vi "Send Command.vi"(7 "Config offset":u64 format="%x", 8 "error in (no error)":errorcluster, 9 "Command payload":u64 format="%x", 10 "Command number":T1, 11 "RP Instrument in":refnum<class "RP Instrument.lvclass">) -> (0 "error out":errorcluster, 3 "RP Instrument out":refnum<class "RP Instrument.lvclass">)   [LabVIEW 2016, in "RP Instrument.lvclass"]
uses:
  RP Instrument.lvclass
  RP Command.ctl
  RP Instrument.lvclass/RP Instrument.ctl
  RP Communicator/RP Communicator.lvclass
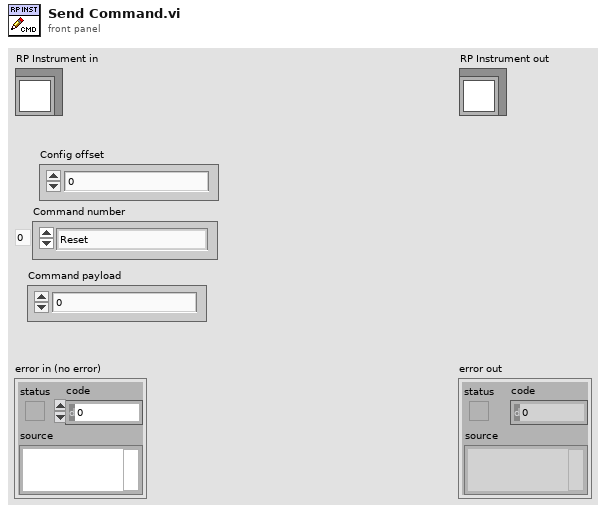
[diagram p1: front panel]
types:
  T1 = typedef "RP Command.ctl" = enum16{"Reset", "Read IDN", "Stop server", "Get status", "Get temperature", "Connect client", "Arm", "Software trigger", "Get whole buffer", "Get chunk", "System call", "Get config", "Set config", "Recieve data", "Recieve Calibartion", "Transmit data"}
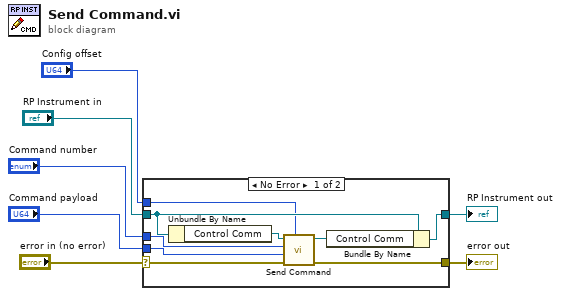
[diagram p0: block diagram]
diagram:
  n1 = case shown="No Error" "error in (no error)" {
    selector: "error in (no error)" -> [w10 w18]
    tunnel: [w9 w18] -> w6
    tunnel: [w15 w17] -> w4
    tunnel: "RP Instrument in" -> [w16 w17]
    tunnel: "Command number" -> [w13 _]
    tunnel: "Config offset" -> [w12 _]
    tunnel: "Command payload" -> [w11 _]
    frame No Error {
      n2 = Unbundle By Name(w16) -> ("Control Comm"=w14:refnum<class "RP Communicator.lvclass">)
      n3 = call-dynamic "Send Command.vi"("Config offset"=w12, "error in (no error)"=w10, "Command payload"=w11, "Command number"=w13, "RP Communicator in"=w14) -> ("error out"=w9:errorcluster, "RP Communicator out"=w8:refnum<class "RP Communicator.lvclass">)  [unwired: 5 in]
      n4 = Bundle By Name(cluster=w16, "Control Comm"=w8) -> (w15:refnum<class "RP Instrument.lvclass">)
    }
    frame Error {
    }
  }
  "error out" <- w6
  "RP Instrument out" <- w4
